vi "PicoScope5000aExampleRapidBlock.vi"() -> ()   [LabVIEW 2009]
doc: "This example demonstrates how to use the PicoScope Labview library to collect data using rapid block mode"
panel:
  in  "Channel A Settings":T1 {"Bandwidth Limit" items=["Full", "20MHz"]; "Range" items=["10 mV", "20 mV", "50 mV", "100 mV", "200 mV", "500 mV", "1 V", "2 V", "5 V", "10 V", "20 V"]; "Coupling" items=["AC", "DC"]}
  out "Analog Channels":cluster{i32, sgl, "Data (Volts)":dbl[]}[](graph)
  out "Trigger Info":T2(array[cluster])
  out "Trigger Offsets":cluster{u64, sgl}[](array[cluster]) {"?" format="%#_5p"}
  out "Properties Panel":T3 {"Max Total Capture Time Available (sec)" format="%.3p"; "Sample Frequency" format="%.3p"; "Sample Rate" format="%.3p"; "Max Samples Available" format="%.3p"; "Total Capture Time (sec)" format="%.3p"}
  in  "Rapid Block Acquisition Settings":T4
  in  "Trigger Settings":T5 {"Trigger Direction" items=["Rising", "Falling"]}
  out "2-channel USB 3.0 device on non-USB 3.0 Port":bool
  out "4-channel USB Powered":bool
  in  "Serial Number":string
  in  "Open using Serial Number":bool
  in  "Resolution":i32(ring) items=["8-bit", "12-bit", "14-bit", "15-bit (max. 2 ch.)", "16-bit (max. 1 ch.)"]
  out "Capture Complete":bool
  in  "Run":bool
  in  "Capture Index":i16 min=0
  in  "stop":bool
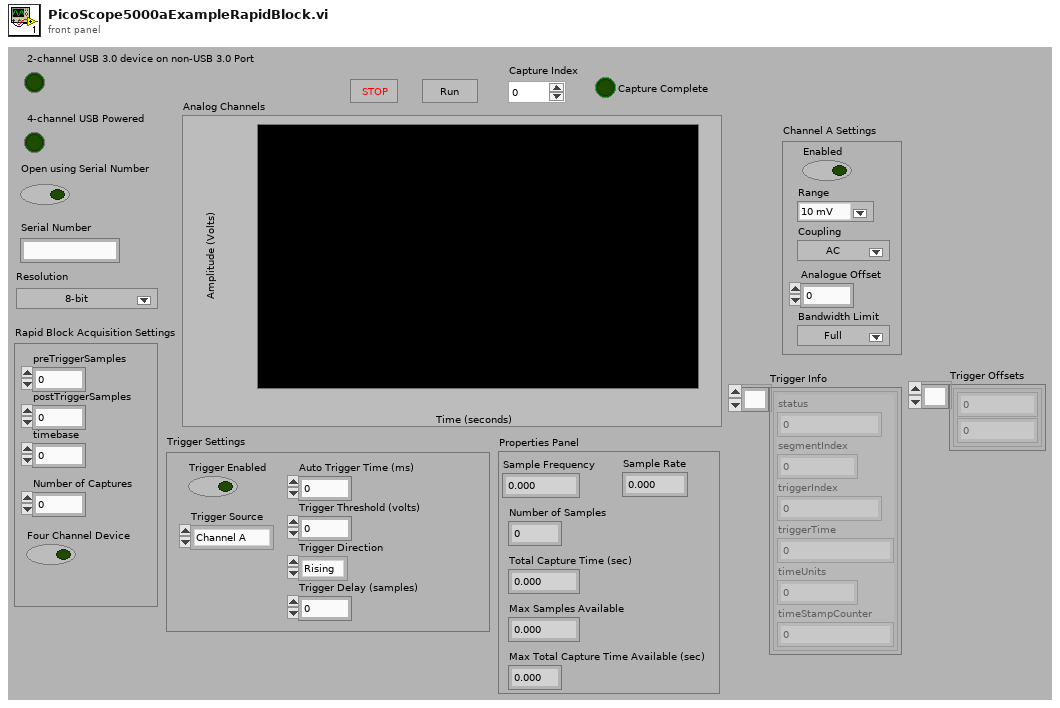
[diagram p1: front panel]
types:
  T1 = cluster{"Enabled":bool, "Coupling":i16, "Range":u16, "Analogue Offset":sgl, "Bandwidth Limit":u32}
  T2 = cluster{"status":u32, "segmentIndex":u32, "triggerIndex":u32, "triggerTime":i64, "timeUnits":i16, "timeStampCounter":u64}[]
  T3 = cluster{"Sample Frequency":sgl, "Sample Rate":sgl, "Max Samples Available":i32, "Number of Samples":u32, "Total Capture Time (sec) ":sgl, "Max Total Capture Time Available (sec)":sgl}
  T4 = cluster{"preTriggerSamples":i32, "postTriggerSamples":i32, "timebase":u32, "Four Channel Device":bool, "Number of Captures":u32}
  T5 = cluster{"Trigger Enabled":bool, "Trigger Source":enum16{"Channel A", "Channel B", "Channel C", "Channel D", "Ext."}, "Trigger Threshold (volts)":dbl, "Trigger Direction":u16, "Trigger Delay (samples)":u32, "Auto Trigger Time (ms)":i16}
  T6 = cluster{"Driver Version":string, "USB Version":string, "Hardware":string, "Variant":string, "Batch and Serial":string, "Cal Date":string, "Kernel Version":string, "Digital HW Version":string, "Analogue HW Version":string, "MSO":bool, "Number of channels":i16}
  T7 = cluster{"preTriggerSamples":i32, "postTriggerSamples":i32, "timebase":u32, "Down-Sample Mode":i32, "Down Sample Ratio":u32}
  T8 = cluster{i32, "Sample Rate":sgl, "Data (Volts)":dbl[]}
  T9 = cluster{i32, "Sample Rate":sgl, "Data (Volts)":dbl[]}[]
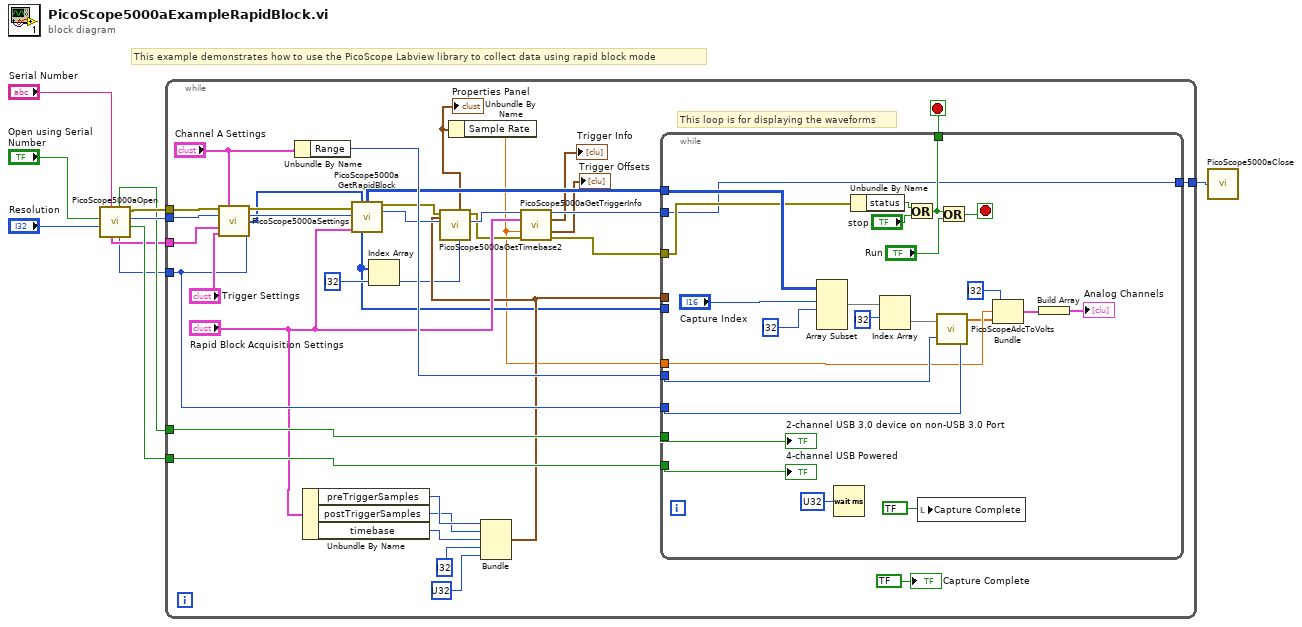
[diagram p0: block diagram]
diagram:
  # "This example demonstrates how to use the PicoScope Labview library to collect data using rapid block mode"
  n1 = call "PicoScope5000aOpen.vi"("Serial Number"="Serial Number", "Resolution"="Resolution", "Use Serial Number"="Open using Serial Number") -> ("USB Powered"=w7:bool, "handle"=w8:i16, "error out"=w9:errorcluster, "Max ADC value"=w1:i16, "USB 3.0 device on non-USB 3.0 Port"=w3:bool, "Device Info"=w2:T6)  [unwired: 3 in]
  n2 = while {
    tunnel: [w27] -> w10
    tunnel: w9 -> [w42]
    tunnel: w8 -> [w41]
    tunnel: w7 -> [w40]
    tunnel: w3 -> [w39]
    tunnel: w2 -> [w37]
    tunnel: w1 -> [w36]
    stop <- w46 stop-if-true
    # "This loop is for displaying the waveforms"
    n3 = call "PicoScope5000aSettings.vi"("error in"=w42, "Channel A Settings"="Channel A Settings", "handle in"=w41, "Device Info"=w37, "Trigger Settings"="Trigger Settings", "Max ADC value"=w36) -> ("error out"=w43:errorcluster, "handle out"=w44:i16, "enabled array"=w34:i16[])  [unwired: 7 in]
    n4 = Unbundle By Name("Channel A Settings") -> ("Range"=w35:u16)
    n5 = Unbundle By Name("Rapid Block Acquisition Settings") -> ("preTriggerSamples"=w32:i32, "postTriggerSamples"=w31:i32, "timebase"=w30:u32)
    n6 = call "PicoScope5000aGetRapidBlock.vi"("error in"=w43, "enabled array"=w34, "handle in"=w44, "Rapid Block Acquisition Settings"="Rapid Block Acquisition Settings") -> ("Channel A Buffer"=w33:i16[][], "error out"=w21:errorcluster, "handle out"=w20:i16, "noOfSamples"=w16:u32[])  [unwired: 3 in, 5 out]
    n7 = Index Array(array=w16, index=i32 ?) -> (element=w17:u32)
    n8 = Bundle("preTriggerSamples"=w32, "postTriggerSamples"=w31, "timebase"=w30, "Down-Sample Mode"=i32 ?, "Down Sample Ratio"=u32 ?) -> (w19:T7)  [unwired: 1 in]
    n9 = call "PicoScope5000aGetTimebase2.vi"("Number of Samples"=w17, "Acquisition Settings"=w19, "handle in"=w20, "error in (no error)"=w21) -> ("handle out"=w23:i16, "error out"=w22:errorcluster, "Properties Panel"=w13:T3)  [unwired: 5 in]
    "Properties Panel" <- w13
    n10 = Unbundle By Name(w13) -> ("Sample Rate"=w12:sgl)
    n11 = call "PicoScope5000aGetTriggerInfo.vi"("handle in"=w23, "Rapid Block Acquisition Settings"="Rapid Block Acquisition Settings", "Sample Rate"=w12, "error in"=w22) -> ("handle out"=w26:i16, "Trigger Info"=→"Trigger Info":T2, "Trigger Offsets"=→"Trigger Offsets":cluster{u64, sgl}[], "error out"=w25:errorcluster)  [unwired: 8 in]
    n12 = while {
      tunnel: [w68] -> w46
      tunnel: w33 -> [w63]
      tunnel: w40 -> [w55]
      tunnel: w39 -> [w56]
      tunnel: w36 -> [w61]
      tunnel: w35 -> [w60]
      tunnel: w26 -> [w52]
      tunnel: w19 -> [_]
      tunnel: [w52] -> w27
      tunnel: w25 -> [w53]
      tunnel: w16 -> [_]
      tunnel: w12 -> [w48]
      stop <- w67 stop-if-true
      n13 = Array Subset(array=w63, index (row)="Capture Index", length (row)=i32 ? ("length")) -> (w59:i16[][])  [unwired: 2 in]
      n14 = Wait (ms)(milliseconds to wait=u32 ?) -> ()  [unwired: 1 out]
      n15 = Unbundle By Name(w53) -> ("status"=w62:bool)
      n16 = Index Array(array=w59, index (row)=i32 ?) -> (element=w57:i16[])  [unwired: 1 in]
      n17 = Or(x=w62, y="stop") -> (x .or. y?=w68:bool)
      n18 = local write "Capture Complete"(bool ? ("Capture Complete")) -> ()
      n19 = call "PicoScopeAdcToVolts.vi"("Max_adc"=w61, "Range Index"=w60, "Data"=w57) -> ("Data (Volts)"=w47:dbl[])
      n20 = Or(x=w68, y="Run") -> (x .or. y?=w67:bool)
      n21 = Bundle(i32 ?, "Sample Rate"=w48, "Data (Volts)"=w47) -> (w50:T8)  [unwired: 1 in]
      n22 = Build Array(w50) -> (→"Analog Channels":T9)
      "2-channel USB 3.0 device on non-USB 3.0 Port" <- w56
      "4-channel USB Powered" <- w55
    }
    "Capture Complete" <- bool ? ("Capture Complete")
  }
  n23 = call "PicoScope5000aClose.vi"("handle"=w10) -> ()
